vi "DifferentPrototype_UseInDLL.vi"(4 "String To Append":string, 5 "Number To Multiply":dbl format="%.2f", 7 "Array In":dbl[](array[numeric]) format="%.2f", 8 "String In":string, 9 "Numeric In":dbl format="%.2f") -> (1 "Array Out":dbl[](array[numeric]) format="%.2f", 2 "String Out":string, 3 "Numeric Out":dbl format="%.2f")   [LabVIEW 2011]
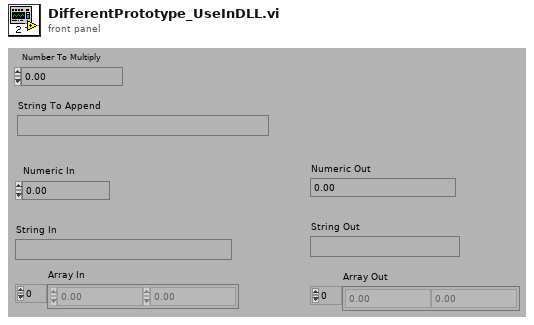
[diagram p1: front panel]
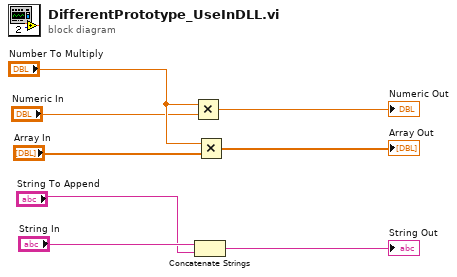
[diagram p0: block diagram]
diagram:
  n1 = Multiply(x="Number To Multiply", y="Numeric In") -> (x*y=→"Numeric Out":dbl)
  n2 = Concatenate Strings("String In", "String To Append") -> (→"String Out":string)
  n3 = Multiply(x="Number To Multiply", y="Array In") -> (x*y=→"Array Out":dbl[])
